vi "Galil_load yield counts.vi"(8 "error in (no error)":errorcluster, 10 "string":dbl, 11 "Programing Logic in":refnum<class "Programing Logic.lvclass">) -> (0 "error out":errorcluster, 3 "Programing Logic out":refnum<class "Programing Logic.lvclass">)   [LabVIEW 2014, in "Programing Logic.lvclass"]
uses:
  Programing Logic.lvclass
  Programing Logic.lvclass/Programing Logic.ctl
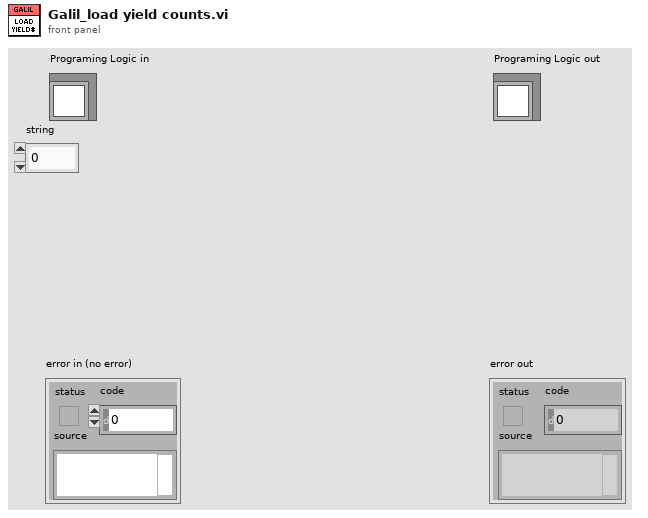
[diagram p1: front panel]
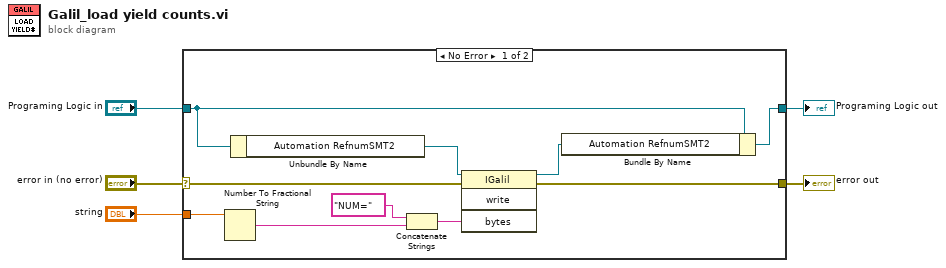
[diagram p0: block diagram]
diagram:
  n1 = case shown="No Error" "error in (no error)" {
    selector: "error in (no error)" -> [w11 w17]
    tunnel: [w10 w17] -> w4
    tunnel: [w14 w16] -> w2
    tunnel: "Programing Logic in" -> [w15 w16]
    tunnel: "string" -> [w7 _]
    frame No Error {
      n2 = Number To Fractional String(number=w7) -> (F-format string=w6:string)  [unwired: 3 in]
      n3 = Unbundle By Name(w15) -> ("Automation RefnumSMT2"=w13:refnum<k7>)
      n4 = Concatenate Strings("NUM=" ("string"), w6) -> (w9:string)
      n5 = invoke class="IGalil" method="write"(reference=w13, error in=w11, "bytes"=w9) -> (reference out=w12:refnum<k7>, error out=w10:errorcluster)  [unwired: 1 in, 2 out]
      n6 = Bundle By Name(cluster=w15, "Automation RefnumSMT2"=w12) -> (w14:refnum<class "Programing Logic.lvclass">)
    }
    frame Error {
    }
  }
  "error out" <- w4
  "Programing Logic out" <- w2
